vi "MICSD Downlink MICS.vi"(8 "Error In":errorcluster, 10 "Downlink":u8[][](array[numeric])=[[1], [255], [255], [255], [1], [0], [0], [0], [0], [0], [0], [0], [0], [0], [255]] format="%02x", 11 "VISA Resource Name":refnum<visa-resource-name>) -> (0 "Error Out":errorcluster, 3 "dup VISA Resource Name":refnum<visa-resource-name>)   [LabVIEW 2020]
panel:
  # "DOWNLINK"
  # "Block 1"
  # "Block 2"
  # "Block 3"
  # "Block 4"
  # "b1"
  # "b2"
  # "b3"
  # "b4"
  # "b5"
  # "b6"
  # "b7"
  # "b8"
  # "b9"
  # "b10"
  # "b11"
  # "b12"
  # "b13"
  # "b14"
  # "b15"
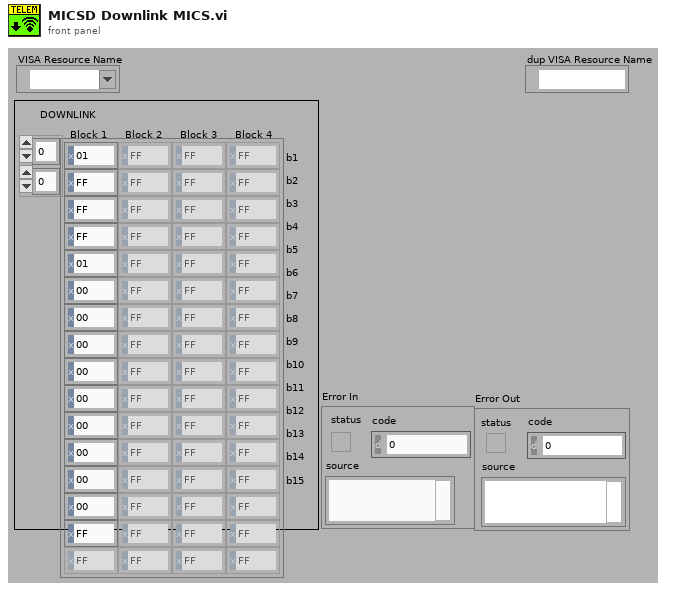
[diagram p1: front panel]
types:
  T1 = cluster{"[0]":i32, "[1]":i32, "[2]":i32, "[3]":i32, "[4]":i32, "[5]":i32, "[6]":i32, "[7]":i32, "[8]":i32}
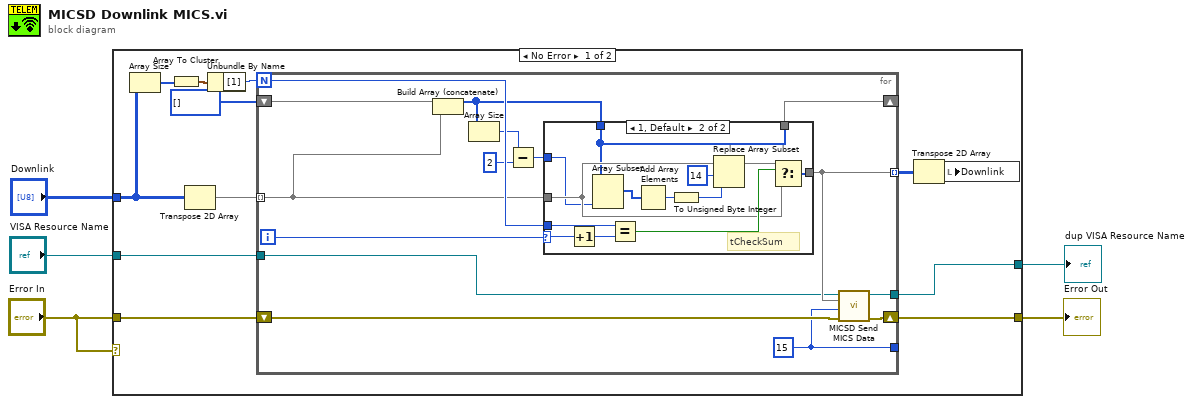
[diagram p0: block diagram]
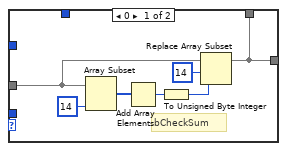
[diagram p2: hidden frame]
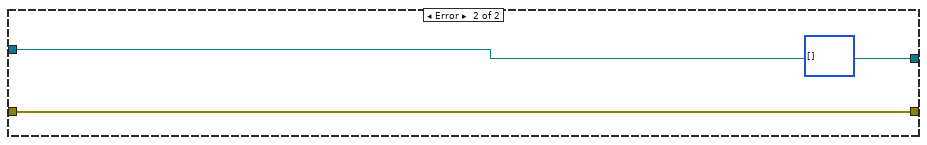
[diagram p3: hidden frame]
diagram:
  n1 = case shown="No Error" "Error In" {
    tunnel: "Downlink" -> [w14 _]
    tunnel: "Error In" -> [w13 w54]
    tunnel: "VISA Resource Name" -> [w12 w53]
    tunnel: [w8 w54] -> w4
    tunnel: [w6 w53] -> w1
    frame No Error {
      n2 = Array Size(array=w14) -> (size(s)=w17:i32[])
      n3 = Array To Cluster(array=w17) -> (cluster=w16:T1)
      n4 = Transpose 2D Array(2D array=w14) -> (transposed array=w11:u8[][])
      n5 = Unbundle By Name(w16) -> ("[1]"=w15:i32)
      n6 = for {
        N: w15 -> [w32]
        tunnel: w11 -> [w26] mode=indexing
        shift-right: [w22] -> w8
        shift-left: w13 -> [w23]
        tunnel: w12 -> [w19]
        tunnel: [w20] -> _
        tunnel: [w21] -> w10 mode=indexing
        shift-right: [w24] -> _
        shift-left: u8[] [] -> [w31]
        tunnel: [w18] -> w6
        i -> [w27]
        w20 = u32 15 ("nBytes")
        n7 = Build Array (concatenate)(w31, w26) -> (w25:u8[])
        n8 = Array Size(array=w25) -> (size(s)=w30:i32)
        n9 = Subtract(x=w30, y=2) -> (x-y=w28:i32)
        n10 = case shown="1, Default" w27 {
          selector: w27 -> [_ w49]
          tunnel: w26 -> [w38 w45]
          tunnel: [w33 w46] -> w21
          tunnel: w32 -> [_ w50]
          tunnel: w25 -> [_ w40]
          tunnel: w28 -> [_ w44]
          tunnel: [w33 w40] -> w24
          frame 0 {
            # "bCheckSum"
            n11 = Array Subset(array=w38, length=14) -> (w36:u8[])  [unwired: 1 in]
            n12 = Add Array Elements(numeric array=w36) -> (sum=w35:u8)
            n13 = To Unsigned Byte Integer(number=w35) -> (unsigned 8bit integer=w34:u8)
            n14 = Replace Array Subset(array=w38, new element=w34, index=14) -> (w33:u8[])
          }
          frame 1, Default {
            # "tCheckSum"
            n15 = Increment(x=w49) -> (x+1=w51:i32)
            n16 = Array Subset(array=w40, length=w44) -> (w42:u8[])  [unwired: 1 in]
            n17 = Equal?(x=w50, y=w51) -> (x = y?=w48:bool)
            n18 = Add Array Elements(numeric array=w42) -> (sum=w43:u8)
            n19 = To Unsigned Byte Integer(number=w43) -> (unsigned 8bit integer=w41:u8)
            n20 = Replace Array Subset(array=w45, new element=w41, index=14) -> (w47:u8[])
            n21 = Select(t=w47, s=w48, f=w45) -> (s? t:f=w46:u8[])
          }
        }
        n22 = call "MICSD Send MICS Data.vi"("error in (no error)"=w23, "BlockSize"=w20, "Send Data"=w21, "VISA Resource Name"=w19) -> ("error out"=w22:errorcluster, "dup VISA Resource Name"=w18:refnum<visa-resource-name>)  [unwired: 6 in]
      }
      n23 = Transpose 2D Array(2D array=w10) -> (transposed array=w9:u8[][])
      n24 = local write "Downlink"(w9) -> ()
    }
    frame Error {
      (unwired) u8[][] [] ("buf")
    }
  }
  "Error Out" <- w4
  "dup VISA Resource Name" <- w1
